vi "FPGA (Top Level).vi"() -> ()   [LabVIEW 2017]
uses:
  <vilib>/LabVIEW Targets/FPGA/cRIO/cRIO-9505/controls.llb/_nicrio_cRIO-9505_DriveStatus.ctl
  <vilib>/Platform/TimedLoop/XDataNode/timing_clust.ctl
  <vilib>/Platform/TimedLoop/XDataNode/nitl_modes.ctl
  <vilib>/Platform/TimedLoop/XDataNode/wakeup.ctl
  <vilib>/rvi/FXPMathLib/FxpSinAndCos/subVIs/nifxpmath_SinAndCos_SimConfig.ctl
  <vilib>/rvi/Emulation/niFpgaGetClockAttributes.vi
  <vilib>/rvi/Emulation/niFpgaSctlEmulationGetInTimedLoop.vi
  <vilib>/rvi/Emulation/niFpgaEmulationReportErrorSimple.vi
  <vilib>/rvi/eio/common/nirviEmuTemplateMethod_errors.vi
  <vilib>/rvi/Emulation/niFpgaEmulationIsFPGAContextNoSignature.vi
  <vilib>/rvi/DataTransferAndStorage/Container/Common/niFpgaContainerGetUniqueNameForEmu.vi
  <vilib>/rvi/Memory/Memory_Emulation/niFpgaMemoryEmulationCacheClearOnFirstRun.vi
  <vilib>/rvi/Memory/Memory_Emulation/nirvimemoryEmulationManagerCache_MakeExclusive.vi
  <vilib>/rvi/Memory/Memory_Emulation/niFpgaMemoryEmulationValidateCache.vi
  <vilib>/rvi/Memory/Memory_Emulation/nirvimemoryEmulationManagerCache_InsertValue.vi
  <vilib>/Utility/error.llb/Clear Errors.vi
  <vilib>/rvi/Memory/Memory_Emulation/nirvimemoryEmulationManagerCache_ReleaseExclusive.vi
  <vilib>/rvi/Memory/Memory_Emulation/nirvimemoryEmulationManagerCache_GetValue.vi
  <vilib>/rvi/Memory/Memory_Emulation/nirvimemoryEmulationManagerCache_SetValue.vi
  <vilib>/rvi/Emulation/niFpgaProcessEmulError.vi
  <vilib>/rvi/Emulation/niFpgaCriticalErrorInLSC.vi
  <vilib>/rvi/FXPMathLib/FxpSinAndCos/simVIs/DllFxpSinAndCosTemp_sub.vi
  <vilib>/eio/EIONode/EIONode.xnode
  <vilib>/rvi/DataTransferAndStorage/Container/XNode/niFpgaContainer.xnode
  <vilib>/rvi/DataTransferAndStorage/Register/Emulation/niFpgaRegisterEmulation.vi
  <vilib>/rvi/FXPMathLib/FxpSinAndCos/XNode/nifxpmath_SinAndCos.xnode
  <vilib>/Platform/TimedLoop/XDataNode/XDataNode.xnode
  <vilib>/Platform/TimedLoop/XDataNode/XDNodeRunTimeDep.lvlib
panel:
  out "Angle 2 (Pi rad)":fxp<+/-,64,16>
  out "Angle 1 (Pi rad)":fxp<+/-,64,17>
  out "x*y 2":fxp<+/-,63,24>
  out "x*y":fxp<+/-,63,24>
  in  "Boolean":bool
  out "Angle 2 (rad)":fxp<+/-,13,4>
  out "Angle 1 (rad)":fxp<+/-,13,4>
  out "Angle 2 (deg)":fxp<+/-,15,10>
  out "Angle 1 (deg)":fxp<+/-,15,10>
  out "Counts 2":i32
  out "Counts 1":i32
  out "PWM Period (ticks)":u32
  out "Link 2 PWM Duty (Counts)":i32
  out "Link 1 PWM Duty (Counts)":i32
  in  "PWM Gen Period (ms)":u16=10
  in  "PWM Period Loops":i32=200
  in  "Link_1 Duty":fxp<+/-,32,0>
  in  "Link_2 Duty":fxp<+/-,32,0>
  in  "LINK1_DRIVE_ENABLED":bool
  in  "LINK2_DRIVE_ENABLED":bool
  out "LINK2_DRIVE_STATUS":T1
  out "LINK1_DRIVE_STATUS":T1
  in  "LINK1_LENGTH_MM":fxp<+,16,12>=2.0 format="%#_19g"
  in  "LINK2_LENGTH_MM":fxp<+,16,12>=2.0 format="%#_19g"
  in  "X_OFFSET_MM":fxp<+/-,33,15>
  in  "Y_OFFSET_MM":fxp<+/-,33,15>
  out "LINK2_Y_MM":fxp<+/-,34,16>
  out "LINK2_X_MM":fxp<+/-,34,16>
  out "LINK1_Y_MM":fxp<+/-,34,16>
  out "LINK1_X_MM":fxp<+/-,34,16>
  out "LINK1_ENC_POS":i32
  out "LINK2_ENC_POS":i32
  out "LINK1_POT_POS":i32
  out "LINK2_POT_POS":i32
  in  "LINK1_ENC_SCALE":fxp<+,32,0> format="%#_32g"
  in  "LINK2_ENC_SCALE":fxp<+,32,0>=0.029296900611370802 format="%#_32g"
  in  "LINK1_PWM_MAX":i16
  in  "LINK2_PWM_MAX":i16
  in  "LINK1_DEMAND_PWM":i16
  in  "LINK2_DEMAND_PWM":i16
  in  "LINK1_POT_SCALE":fxp<+/-,32,16>
  in  "LINK1_OFFSET":fxp<+/-,16,16>
  in  "LINK2_POT_SCALE":fxp<+/-,32,16>
  in  "LINK2_OFFSET":fxp<+/-,16,16>
  in  "AI_POT_LOOP_US":u16=10
  in  "ENC_DEBOUNCE_CYCLES":u16=5
  in  "LINK1_ENC_CNTS":i32
  in  "LINK2_ENC_CNTS":i32
  in  "LINK1_UPDATE_ENC":bool
  in  "LINK2_UPDATE_ENC":bool
  # "PWM at 50kHz"
  # "10MHz Loops Rate"
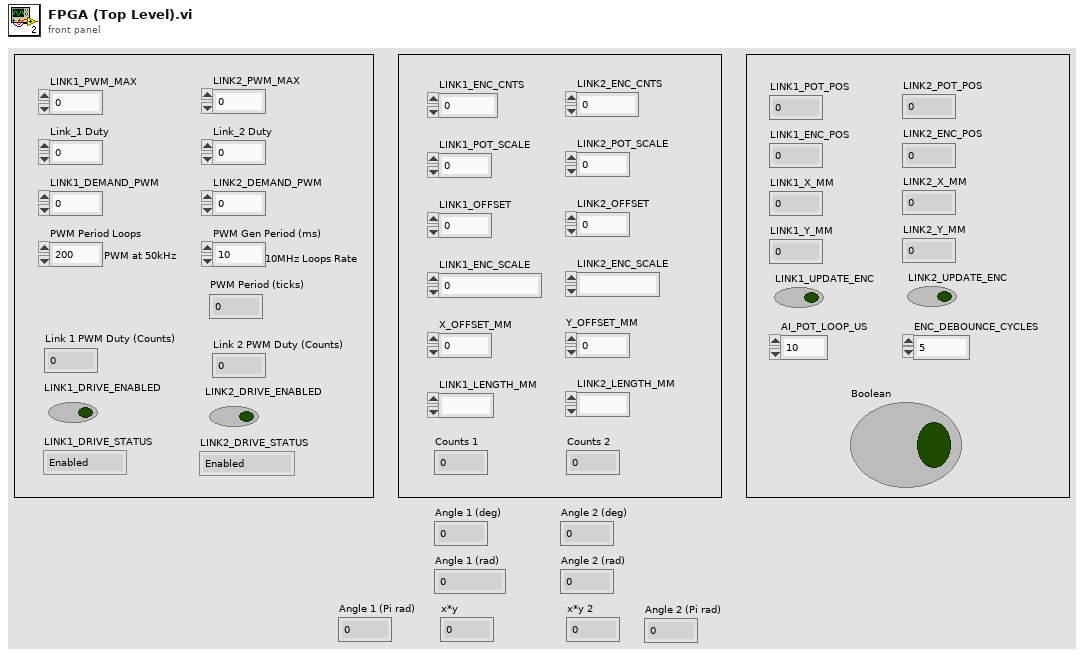
[diagram p1: front panel]
types:
  T1 = typedef "_nicrio_cRIO-9505_DriveStatus.ctl" = enum8{"Enabled", "Disabled", "Disabled by Drive Fault", "Disabled by Temp. Fault", "Disabled by E-Stop", "Unknown"}
  T2 = typedef "XDNodeRunTimeDep.lvlib/timing_clust.ctl" = cluster{"Expected End [f-1]":u64, "Actual End [f-1]":u64, "Finished Late? [f-1]":bool, "Expected End [i-1]":u64, "Actual End [i-1]":u64, "Finished Late? [i-1]":bool, "Expected Start [i]":u64, "Actual Start [i]":u64, "Expected Start [f]":u64, "Actual Start [f]":u64, "Source Name":string, "Structure Name":string, "Period":i64, "Deadline":i64, "Offset":i64, "Start":i64, "Priority":i32, "Timeout":i32, "Mode":T3, "Wakeup Reason":T4, "Error":errorcluster, "Source Type":string, "Secondary Source Type":string, "Global End Time":u64, "Global Start Time":u64, "Frame Duration":u64, "Iteration Duration":u64, "Assigned CPU":i32, "I/O Scan Engine Mode":u32}
  T3 = typedef "XDNodeRunTimeDep.lvlib/nitl_modes.ctl" = enum32{"No Change", "Process missed periods, maintain original phase", "Discard missed periods, maintain original phase", "Process missed periods, ignore original phase", "Discard missed periods, ignore original phase"}
  T4 = typedef "XDNodeRunTimeDep.lvlib/wakeup.ctl" = enum32{"Normal", "Aborted", "Asynchronous wakeup", "Timing source error", "Timed loop error", "Timeout"}
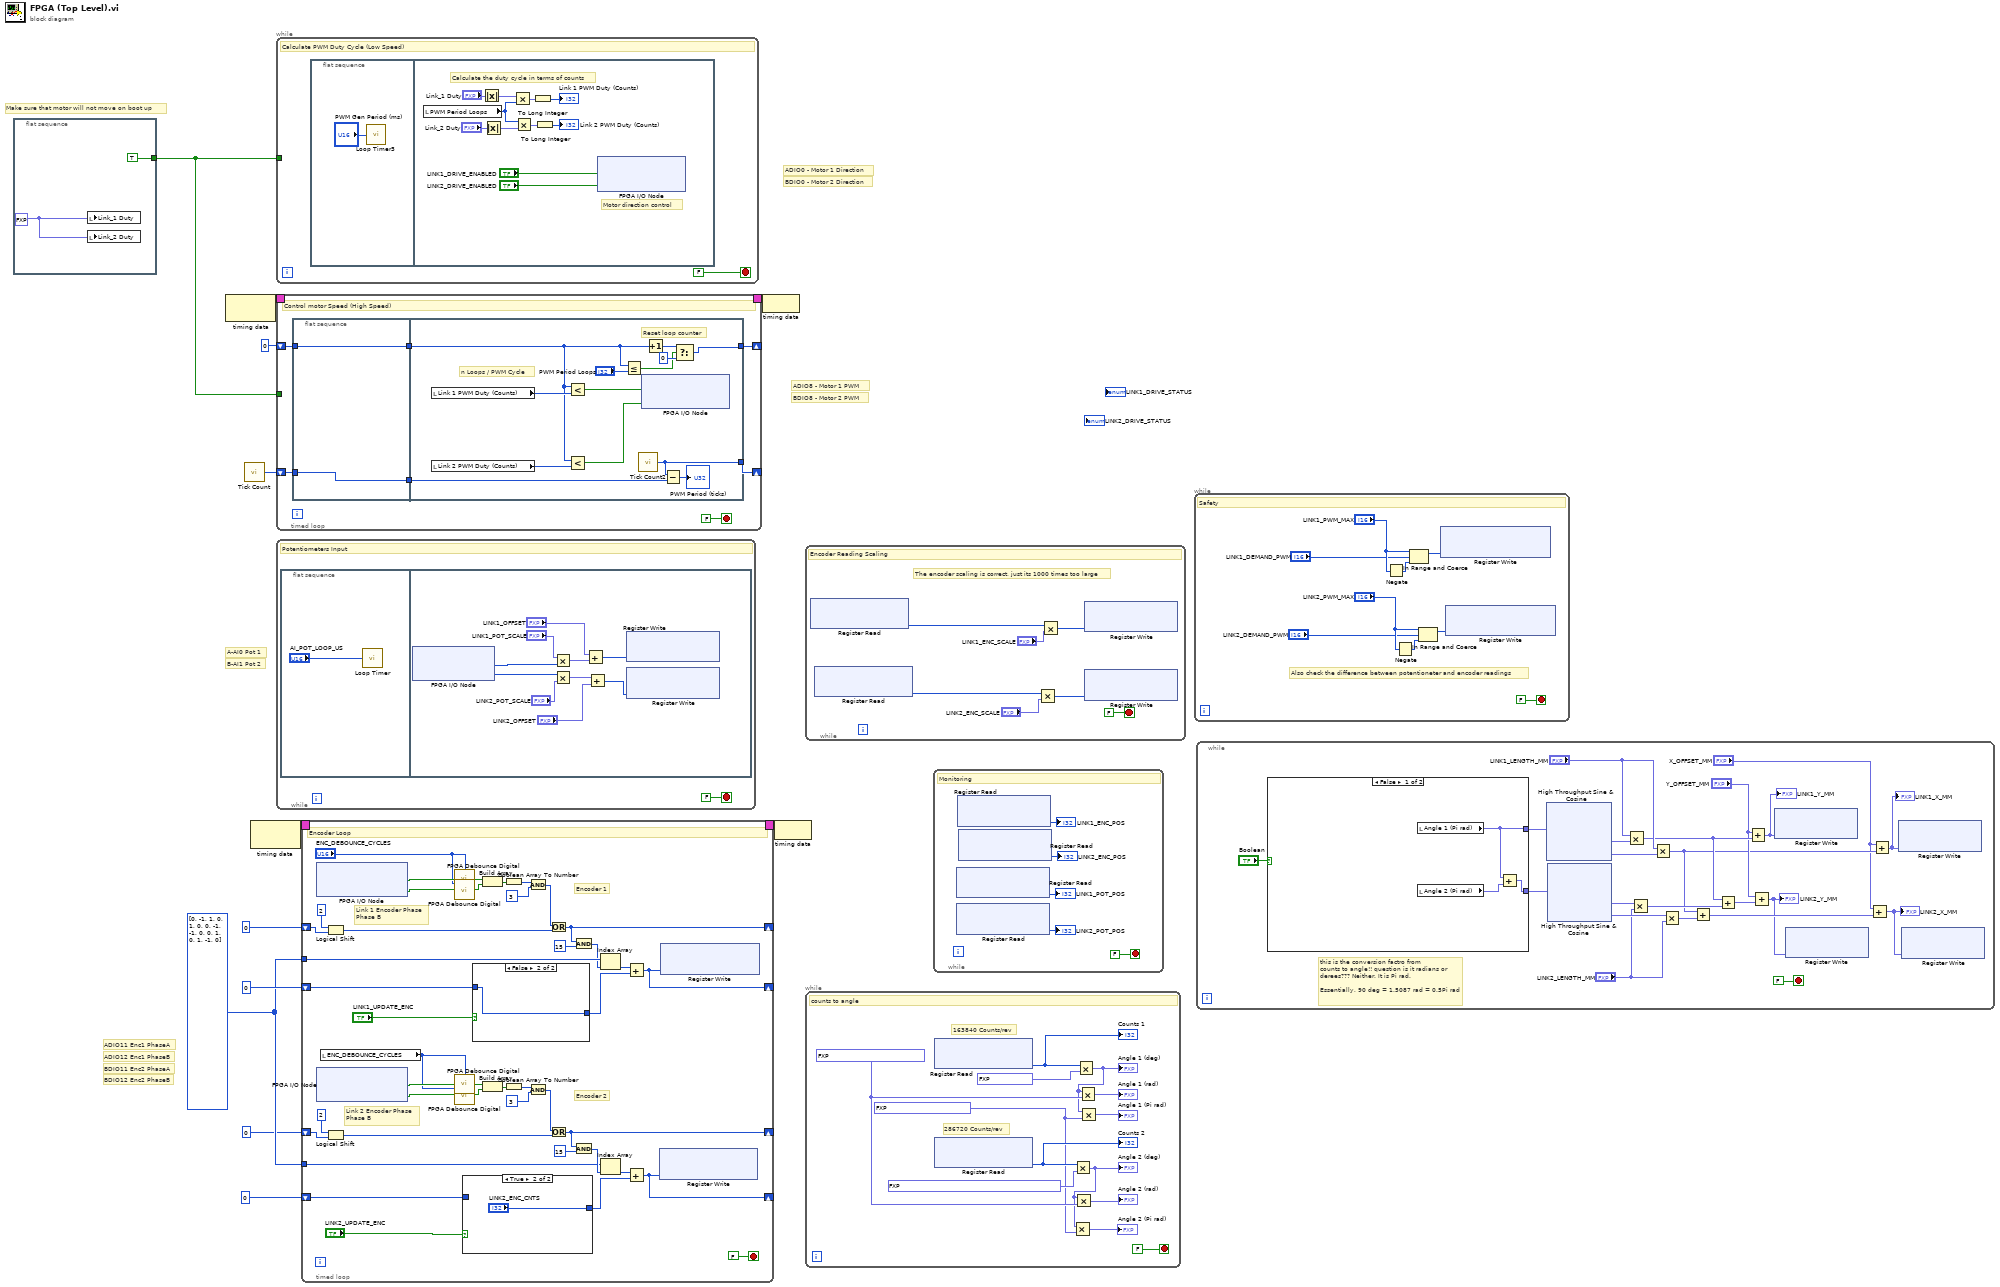
[diagram p0: block diagram]
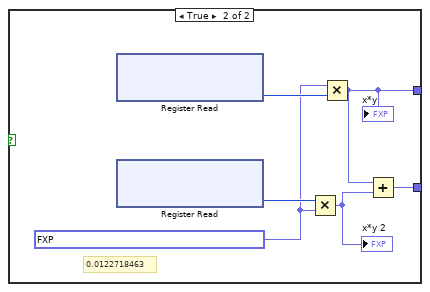
[diagram p2: hidden frame]
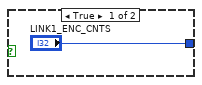
[diagram p4: hidden frame]
diagram:
  w8 = i8[] [0, -1, 1, 0, 1, 0, 0, -1, -1, 0, 0, 1, 0, 1, -1, 0]
  # "BDIO0 - Motor 2 Direction"
  # "ADIO0 - Motor 1 Direction"
  # "BDIO8 - Motor 2 PWM"
  # "ADIO8 - Motor 1 PWM"
  # "B-AI1 Pot 2"
  # "A-AI0 Pot 1"
  # "BDIO12 Enc2 PhaseB"
  # "BDIO11 Enc2 PhaseA"
  # "ADIO12 Enc1 PhaseB"
  # "ADIO11 Enc1 PhaseA"
  # "Make sure that motor will not move on boot up"
  n1 = flat-sequence {
    tunnel: [TRUE] -> w1
    frame #0 {
      w14 = fxp<+/-,32,0> 0.0 ("Link_1 Duty")
      n2 = local write "Link_1 Duty"(w14) -> ()
      n3 = local write "Link_2 Duty"(w14) -> ()
    }
  }
  n4 = node-c288() -> (w4:T2)  [unwired: 1 in]
  n5 = call "Tick Count"() -> ("Tick Count(Ticks)"=w5:u32)
  n6 = node-c288() -> (w12:T2)  [unwired: 1 in]
  n7 = while {
    tunnel: w1 -> [_]
    stop <- FALSE stop-if-true
    # "Calculate PWM Duty Cycle (Low Speed)"
    n8 = flat-sequence {
      frame #0 {
        n9 = call "Loop Timer3"("Count(mSec)"="PWM Gen Period (ms)") -> ()  [unwired: 1 out]
      }
      frame #1 {
        # "Motor direction control"
        # "Calculate the duty cycle in terms of counts"
        n10 = local read "PWM Period Loops"() -> (w21:i32)
        n11 = Absolute Value(x="Link_1 Duty") -> (abs(x)=w25:fxp<+,32,0>)
        n12 = Absolute Value(x="Link_2 Duty") -> (abs(x)=w22:fxp<+,32,0>)
        n13 = Multiply(x=w25, y=w21) -> (x*y=w26:fxp<+/-,63,31>)
        n14 = Multiply(x=w21, y=w22) -> (x*y=w24:fxp<+/-,63,31>)
        n15 = To Long Integer(number=w26) -> (32bit integer=→"Link 1 PWM Duty (Counts)":i32)
        n16 = To Long Integer(number=w24) -> (32bit integer=→"Link 2 PWM Duty (Counts)":i32)
        n17 = xnode "FPGA I/O Node"("ConnectorA/DIO0"="LINK1_DRIVE_ENABLED", "ConnectorB/DIO0"="LINK2_DRIVE_ENABLED") -> ()  [unwired: 2 in, 2 out]
      }
    }
  }
  n18 = timed-loop {
    shift-right: [w33] -> _
    shift-left: w5 -> [w32]
    timing: w4 -> [_]
    timing-out: [_] -> w3
    shift-right: [w30] -> _
    shift-left: i16 0 -> [w29]
    tunnel: w1 -> [_]
    stop <- FALSE stop-if-true
    # "Control motor Speed (High Speed)"
    n19 = flat-sequence {
      tunnel: w32 -> [w36]
      tunnel: [w36] -> w31
      tunnel: w29 -> [w35]
      tunnel: [w35] -> w28
      tunnel: [w45] -> w33
      tunnel: w31 -> [w44]
      tunnel: [w41] -> w30
      tunnel: w28 -> [w38]
      frame #0 {
      }
      frame #1 {
        # "Reset loop counter"
        # "n Loops / PWM Cycle"
        n20 = local read "Link 1 PWM Duty (Counts)"() -> (w47:i32)
        n21 = local read "Link 2 PWM Duty (Counts)"() -> (w46:i32)
        n22 = Less?(x=w38, y=w47) -> (x < y?=w49:bool)
        n23 = Less?(x=w38, y=w46) -> (x < y?=w48:bool)
        n24 = Less Or Equal?(x=w38, y="PWM Period Loops") -> (x <= y?=w37:bool)
        n25 = call "Tick Count2"() -> ("Tick Count(Ticks)"=w45:u32)
        n26 = xnode "FPGA I/O Node"("ConnectorA/DIO8"=w49, "ConnectorB/DIO8"=w48) -> ()  [unwired: 2 in, 2 out]
        n27 = Increment(x=w38) -> (x+1=w42:i16)
        n28 = Subtract(x=w45, y=w44) -> (x-y=→"PWM Period (ticks)":u32)
        n29 = Select(t=w42, s=w37, f=i16 0) -> (s? t:f=w41:i16)
      }
    }
  }
  n30 = while {
    stop <- FALSE stop-if-true
    # "Potentiometers Input"
    n31 = flat-sequence {
      frame #0 {
        n32 = call "Loop Timer"("Count(uSec)"="AI_POT_LOOP_US") -> ()  [unwired: 1 out]
      }
      frame #1 {
        n33 = xnode "FPGA I/O Node"() -> ("ConnectorA/AI0"=w55:u16, "ConnectorB/AI1"=w54:u16)  [unwired: 2 in, 2 out]
        n34 = Multiply(x="LINK1_POT_SCALE", y=w55) -> (x*y=w62:fxp<+/-,48,32>)
        n35 = Multiply(x=w54, y="LINK2_POT_SCALE") -> (x*y=w58:fxp<+/-,48,32>)
        n36 = Add(x="LINK1_OFFSET", y=w62) -> (x+y=w56:i32)
        n37 = Add(x=w58, y="LINK2_OFFSET") -> (x+y=w57:i32)
        n38 = xnode ("Register Write")("Data"=w56) -> ()  [unwired: 1 in, 1 out]
        n39 = xnode ("Register Write")("Data"=w57) -> ()  [unwired: 1 in, 1 out]
      }
    }
  }
  n40 = timed-loop {
    timing: w12 -> [_]
    timing-out: [_] -> w11
    tunnel: w8 -> [w103]
    shift-right: [w96] -> _
    shift-left: u8 0 -> [w105]
    shift-right: [w67] -> _
    shift-left: 0 -> [w88]
    tunnel: w8 -> [w72]
    shift-right: [w70] -> _
    shift-left: u8 0 -> [w71]
    shift-right: [w66] -> _
    shift-left: 0 -> [w64]
    stop <- FALSE stop-if-true
    # "Link 2 Encoder Phase \nPhase B"
    # "Link 1 Encoder Phase \nPhase B"
    # "Encoder 2"
    # "Encoder 1"
    # "Encoder Loop"
    n41 = xnode "FPGA I/O Node"() -> ("ConnectorA/DIO11"=w94:bool, "ConnectorA/DIO12"=w93:bool)  [unwired: 2 in, 2 out]
    n42 = xnode "FPGA I/O Node"() -> ("ConnectorB/DIO11"=w78:bool, "ConnectorB/DIO12"=w77:bool)  [unwired: 2 in, 2 out]
    n43 = local read "ENC_DEBOUNCE_CYCLES"() -> (w69:u16)
    n44 = Logical Shift(y=i16 2, x=w105) -> (x << y=w98:u8)
    n45 = Logical Shift(y=i16 2, x=w71) -> (x << y=w81:u8)
    n46 = call "FPGA Debounce Digital.vi"("Input Signal"=w94, "Cycles to Filter"="ENC_DEBOUNCE_CYCLES") -> ("Output Filtered Signal"=w92:bool)
    n47 = call "FPGA Debounce Digital.vi"("Input Signal"=w93, "Cycles to Filter"="ENC_DEBOUNCE_CYCLES") -> ("Output Filtered Signal"=w91:bool)
    n48 = call "FPGA Debounce Digital.vi"("Input Signal"=w78, "Cycles to Filter"=w69) -> ("Output Filtered Signal"=w76:bool)
    n49 = call "FPGA Debounce Digital.vi"("Input Signal"=w77, "Cycles to Filter"=w69) -> ("Output Filtered Signal"=w75:bool)
    n50 = case shown="True" "LINK2_UPDATE_ENC" {
      tunnel: w64 -> [w107 _]
      tunnel: [w107 "LINK2_ENC_CNTS"] -> w73
      frame False {
      }
      frame True {
      }
    }
    n51 = case shown="False" "LINK1_UPDATE_ENC" {
      tunnel: w88 -> [_ w110]
      tunnel: ["LINK1_ENC_CNTS" w110] -> w87
      frame True {
      }
      frame False {
      }
    }
    n52 = Build Array(w92, w91) -> (w90:bool[])
    n53 = Build Array(w76, w75) -> (w74:bool[])
    n54 = Boolean Array To Number(Boolean array=w90) -> (number=w101:u8)
    n55 = Boolean Array To Number(Boolean array=w74) -> (number=w84:u8)
    n56 = And(x=w101, y=u8 3) -> (x .and. y?=w99:u8)
    n57 = And(x=w84, y=u8 3) -> (x .and. y?=w82:u8)
    n58 = Or(x=w99, y=w98) -> (x .or. y?=w96:u8)
    n59 = Or(x=w82, y=w81) -> (x .or. y?=w70:u8)
    n60 = And(x=w96, y=u8 15) -> (x .and. y?=w97:u8)
    n61 = And(x=w70, y=u8 15) -> (x .and. y?=w80:u8)
    n62 = Index Array(array=w103, index=w97) -> (element=w95:i8)
    n63 = Index Array(array=w72, index=w80) -> (element=w79:i8)
    n64 = Add(x=w95, y=w87) -> (x+y=w67:i32)
    n65 = Add(x=w79, y=w73) -> (x+y=w66:i32)
    n66 = xnode ("Register Write")("Data"=w66) -> ()  [unwired: 1 in, 1 out]
    n67 = xnode ("Register Write")("Data"=w67) -> ()  [unwired: 1 in, 1 out]
  }
  n68 = node-c288(w3) -> ()
  n69 = node-c288(w11) -> ()
  n70 = while {
    stop <- FALSE stop-if-true
    # "The encoder scaling is correct, just its 1000 times too large"
    # "Encoder Reading Scaling"
    n71 = xnode ("Register Read")() -> ("Data"=w117:i32)  [unwired: 1 in, 1 out]
    n72 = xnode ("Register Read")() -> ("Data"=w118:i32)  [unwired: 1 in, 1 out]
    n73 = Multiply(x=w118, y="LINK2_ENC_SCALE") -> (x*y=w115:i32)
    n74 = Multiply(x=w117, y="LINK1_ENC_SCALE") -> (x*y=w116:i32)
    n75 = xnode ("Register Write")("Data"=w116) -> ()  [unwired: 1 in, 1 out]
    n76 = xnode ("Register Write")("Data"=w115) -> ()  [unwired: 1 in, 1 out]
  }
  n77 = while {
    stop <- FALSE stop-if-true
    w121 = fxp<+,15,-7> 0.005555629730224609
    w125 = fxp<+,21,-5> 0.017453297972679138
    # "286720 Counts/rev"
    # "163840 Counts/rev"
    # "counts to angle"
    n78 = xnode ("Register Read")() -> ("Data"=w129:i32)  [unwired: 1 in, 1 out]
    "Counts 1" <- w129
    n79 = xnode ("Register Read")() -> ("Data"=w127:i32)  [unwired: 1 in, 1 out]
    "Counts 2" <- w127
    n80 = Multiply(x=w127, y=fxp<+,35,-9> 0.0012555803569966884) -> (x*y=w122:fxp<+/-,64,23>)
    "Angle 2 (deg)" <- w122
    n81 = Multiply(x=w122, y=w121) -> (x*y=→"Angle 2 (Pi rad)":fxp<+/-,64,16>)
    n82 = Multiply(x=w122, y=w125) -> (x*y=→"Angle 2 (rad)":fxp<+/-,64,18>)
    n83 = Multiply(x=w129, y=fxp<+,35,-8> 0.002197265625) -> (x*y=w124:fxp<+/-,64,24>)
    "Angle 1 (deg)" <- w124
    n84 = Multiply(x=w124, y=w125) -> (x*y=→"Angle 1 (rad)":fxp<+/-,64,19>)
    n85 = Multiply(x=w124, y=w121) -> (x*y=→"Angle 1 (Pi rad)":fxp<+/-,64,17>)
  }
  n86 = while {
    stop <- FALSE stop-if-true
    # "Monitoring"
    n87 = xnode ("Register Read")() -> ("Data"=→"LINK1_POT_POS":i32)  [unwired: 1 in, 1 out]
    n88 = xnode ("Register Read")() -> ("Data"=→"LINK2_POT_POS":i16)  [unwired: 1 in, 1 out]
    n89 = xnode ("Register Read")() -> ("Data"=→"LINK1_ENC_POS":i32)  [unwired: 1 in, 1 out]
    n90 = xnode ("Register Read")() -> ("Data"=→"LINK2_ENC_POS":i32)  [unwired: 1 in, 1 out]
  }
  n91 = while {
    stop <- FALSE stop-if-true
    # "Also check the difference between potentioneter and encoder readings"
    # "Safety"
    n92 = Negate(x="LINK1_PWM_MAX") -> (-x=w144:i16)
    n93 = Negate(x="LINK2_PWM_MAX") -> (-x=w142:i16)
    n94 = In Range and Coerce(upper limit="LINK1_PWM_MAX", x="LINK1_DEMAND_PWM", lower limit=w144) -> (coerced(x)=w145:i16)  [unwired: 1 out]
    n95 = In Range and Coerce(upper limit="LINK2_PWM_MAX", x="LINK2_DEMAND_PWM", lower limit=w142) -> (coerced(x)=w141:i16)  [unwired: 1 out]
    n96 = xnode ("Register Write")("Data"=w145) -> ()  [unwired: 1 in, 1 out]
    n97 = xnode ("Register Write")("Data"=w141) -> ()  [unwired: 1 in, 1 out]
  }
  n98 = while {
    stop <- FALSE stop-if-true
    # "this is the conversion factro from \ncounts to angle!! question is it radians or\nderees??? Neither. It is Pi rad. \n\nEssentially, 90 deg = 1.5087 rad = 0.5Pi rad"
    n99 = case shown="False" "Boolean" {
      tunnel: [w169 w177] -> w167
      tunnel: [w171 w176] -> w148
      frame False {
        n100 = local read "Angle 1 (Pi rad)"() -> (w171:fxp<+/-,64,17>)
        n101 = local read "Angle 2 (Pi rad)"() -> (w170:fxp<+/-,64,16>)
        n102 = Add(x=w171, y=w170) -> (x+y=w169:fxp<+/-,64,18>)
      }
      frame True {
        w173 = fxp<+,31,-8> 5.555555617320351e-05
        # "0.0122718463"
        n103 = xnode ("Register Read")() -> ("Data"=w174:i32)  [unwired: 1 in, 1 out]
        n104 = xnode ("Register Read")() -> ("Data"=w175:i32)  [unwired: 1 in, 1 out]
        n105 = Multiply(x=w175, y=w173) -> (x*y=w172:fxp<+/-,63,24>)
        "x*y 2" <- w172
        n106 = Multiply(x=w173, y=w174) -> (x*y=w176:fxp<+/-,63,24>)
        "x*y" <- w176
        n107 = Add(x=w176, y=w172) -> (x+y=w177:fxp<+/-,64,25>)
      }
    }
    n108 = xnode "High Throughput Sine & Cosine"("x (pi)"=w148) -> ("sin(x)"=w166:fxp<+/-,16,2>, "cos(x)"=w165:fxp<+/-,16,2>)
    n109 = xnode "High Throughput Sine & Cosine"("x (pi)"=w167) -> ("sin(x)"=w163:fxp<+/-,16,2>, "cos(x)"=w162:fxp<+/-,16,2>)
    n110 = Multiply(x="LINK1_LENGTH_MM", y=w166) -> (x*y=w158:fxp<+/-,32,14>)
    n111 = Multiply(x=w163, y="LINK2_LENGTH_MM") -> (x*y=w159:fxp<+/-,32,14>)
    n112 = Multiply(x="LINK1_LENGTH_MM", y=w165) -> (x*y=w155:fxp<+/-,32,14>)
    n113 = Multiply(x=w162, y="LINK2_LENGTH_MM") -> (x*y=w160:fxp<+/-,32,14>)
    n114 = Add(x=w155, y=w160) -> (x+y=w154:fxp<+/-,33,15>)
    n115 = Add(x=w158, y=w159) -> (x+y=w157:fxp<+/-,33,15>)
    n116 = Add(x="Y_OFFSET_MM", y=w158) -> (x+y=w150:fxp<+/-,34,16>)
    "LINK1_Y_MM" <- w150
    n117 = Add(x="Y_OFFSET_MM", y=w157) -> (x+y=w152:fxp<+/-,34,16>)
    "LINK2_Y_MM" <- w152
    n118 = xnode ("Register Write")("Data"=w150) -> ()  [unwired: 1 in, 1 out]
    n119 = xnode ("Register Write")("Data"=w152) -> ()  [unwired: 1 in, 1 out]
    n120 = Add(x="X_OFFSET_MM", y=w154) -> (x+y=w151:fxp<+/-,34,16>)
    "LINK2_X_MM" <- w151
    n121 = Add(x="X_OFFSET_MM", y=w155) -> (x+y=w149:fxp<+/-,34,16>)
    "LINK1_X_MM" <- w149
    n122 = xnode ("Register Write")("Data"=w149) -> ()  [unwired: 1 in, 1 out]
    n123 = xnode ("Register Write")("Data"=w151) -> ()  [unwired: 1 in, 1 out]
  }
